vi "from string.vi"(8 "error in":errorcluster, 9 "data":string, 10 "version":string, 11 "EthernetIP configuration in":refnum<class "EthernetIP configuration.lvclass">) -> (0 "error out":errorcluster, 3 "EthernetIP configuration out":refnum<class "EthernetIP configuration.lvclass">)   [LabVIEW 2013, in "EthernetIP configuration.lvclass"]
doc: "Provides an interface for loading a module configuration from a file or other serialized data source. It is recommended that all children of this class store data in two sets--data required for its own initialization, and any data required for parent initialization--and that each implementation uses the <b>Call Parent Method</b> primitive to de-serialize parent information. As a result, it is expected that every module configuration class calls <b>component configuration.lvclass:From String.vi</b>."
uses:
  EthernetIP configuration.lvclass
  assembly definition.ctl
  assembly type.ctl
  <vilib>/NI/Tag Bus/tag/Data Type.ctl
  <vilib>/NI/Tag Bus Module Framework/module configuration/TBM module configuration.lvclass
  EthernetIP configuration.lvclass/EthernetIP configuration.ctl
  channel/EthernetIP Channel.lvclass
  <vilib>/NI/Tag Bus Module Framework/root configuration/TBM configuration.lvclass
  <vilib>/NI/Tag Bus/tag/tag descriptor.lvclass
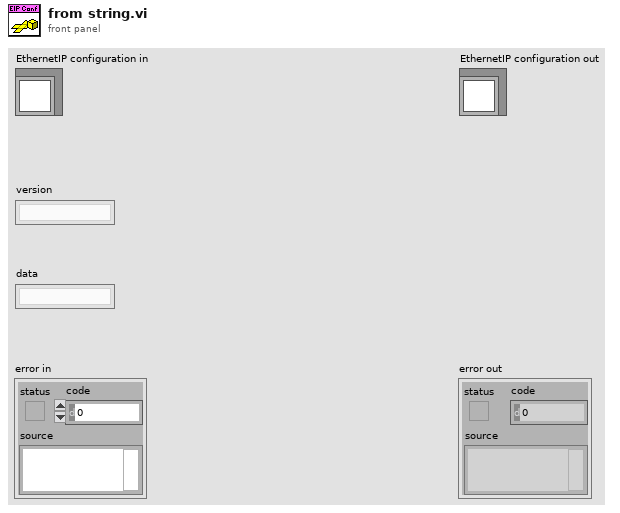
[diagram p1: front panel]
types:
  T1 = typedef "EthernetIP configuration.lvclass/assembly definition.ctl" = cluster{"name":string, "Instance ID":u32, "Type":T2, "Size (elements)":u32, "big endian?":bool, "data type":T3}
  T2 = typedef "EthernetIP configuration.lvclass/assembly type.ctl" = enum32{"Producing", "Consuming"}
  T3 = typedef "tag bus.lvlib/tag descriptor.lvclass/Data Type.ctl" = enum16{"Double", "Single", "I64", "I32", "I16", "I8", "U64", "U32", "U16", "U8", "Boolean", "String", "Array of Double", "Array of Single", "Array of I64", "Array of I32", "Array of I16", "Array of I8", "Array of U64", "Array of U32", "Array of U16", "Array of U8", "Array of Boolean", "Array of String"}
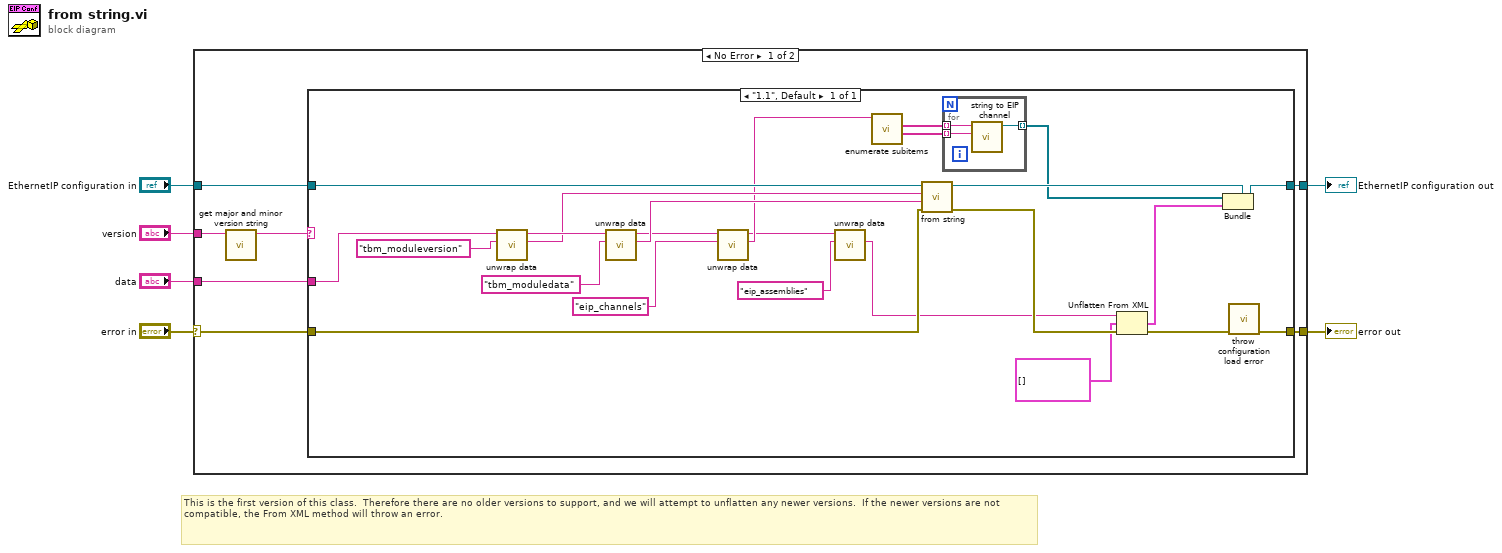
[diagram p0: block diagram]
diagram:
  # "This is the first version of this class.  Therefore there are no older versions to support, and we will attempt to unflatten any newer versions.  If the newer versions are not compatible, the From XML method will throw an error."
  n1 = case shown="No Error" "error in" {
    selector: "error in" -> [w7 w42]
    tunnel: "data" -> [w13 _]
    tunnel: "EthernetIP configuration in" -> [w12 w41]
    tunnel: [w11 w41] -> w5
    tunnel: [w10 w42] -> w4
    tunnel: "version" -> [w9 _]
    frame No Error {
      n2 = call <vilib>:"get major and minor version string.vi"("full version"=w9) -> ("major.minor version"=w8:string)  [unwired: 10 in]
      n3 = case shown="\"1.1\", Default" w8 {
        tunnel: w13 -> [w33]
        tunnel: w7 -> [w32]
        tunnel: w12 -> [w37]
        tunnel: [w27] -> w11
        tunnel: [w35] -> w10
        frame "1.1", Default {
          n4 = call <vilib>:"unwrap data.vi"("identifier"="tbm_moduleversion" ("additional identifier"), "data to unwrap"=w33) -> ("unwrapped data"=w28:string, "remaining string"=w34:string)  [unwired: 8 in]
          n5 = call <vilib>:"unwrap data.vi"("identifier"="tbm_moduledata" ("additional identifier"), "data to unwrap"=w34) -> ("unwrapped data"=w30:string, "remaining string"=w26:string)  [unwired: 8 in]
          n6 = call <vilib>:"unwrap data.vi"("identifier"="eip_channels" ("additional identifier"), "data to unwrap"=w26) -> ("unwrapped data"=w25:string, "remaining string"=w18:string)  [unwired: 8 in]
          n7 = call <vilib>:"unwrap data.vi"("identifier"="eip_assemblies" ("additional identifier"), "data to unwrap"=w18) -> ("unwrapped data"=w17:string)  [unwired: 8 in, 1 out]
          n8 = call <vilib>:"enumerate subitems.vi"("data to enumerate"=w25) -> ("associated data"=w23:string[], "discovered subitems"=w24:string[])  [unwired: 8 in, 1 out]
          n9 = call-parent "from string.vi"("error in"=w32, "data"=w30, "version"=w28, "module configuration in"=w37) -> ("error out"=w21:errorcluster, "module configuration out"=w36:refnum<class "EthernetIP configuration.lvclass">)  [unwired: 6 in]
          n10 = for {
            tunnel: w24 -> [w40] mode=indexing
            tunnel: w23 -> [w39] mode=indexing
            tunnel: [w38] -> w22 mode=indexing
            n11 = call "string to EIP channel.vi"("channel data"=w39, "identifier"=w40) -> ("channel in"=w38:refnum<class "EthernetIP Channel.lvclass">)  [unwired: 9 in]
          }
          n12 = Unflatten From XML(xml string=w17, type=T1[] [] ("assemblies"), error in (no error)=w21) -> (value=w19:T1[], error out=w20:errorcluster)
          n13 = Bundle(cluster=w36, w22, w19) -> (w27:refnum<class "EthernetIP configuration.lvclass">)
          n14 = call <vilib>:"throw configuration load error.vi"("error in"=w20) -> ("error out"=w35:errorcluster)  [unwired: 10 in]
        }
      }
    }
    frame Error {
    }
  }
  "error out" <- w4
  "EthernetIP configuration out" <- w5
